vi "Tree.vi"() -> ()   [LabVIEW 2013]
panel:
  in  "全收回":bool
  in  "全展开":bool
  in  "新建项目":bool
  out "当前油动机":string
  out "当前项目":string
  in  "新建油动机":bool
  in  "刷新":bool
  in  "stop":bool
  in  "Path":path
  in  "Tree":string(tree)
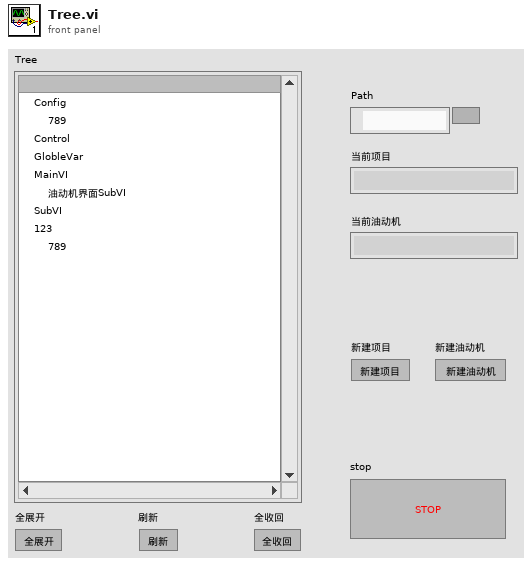
[diagram p1: front panel]
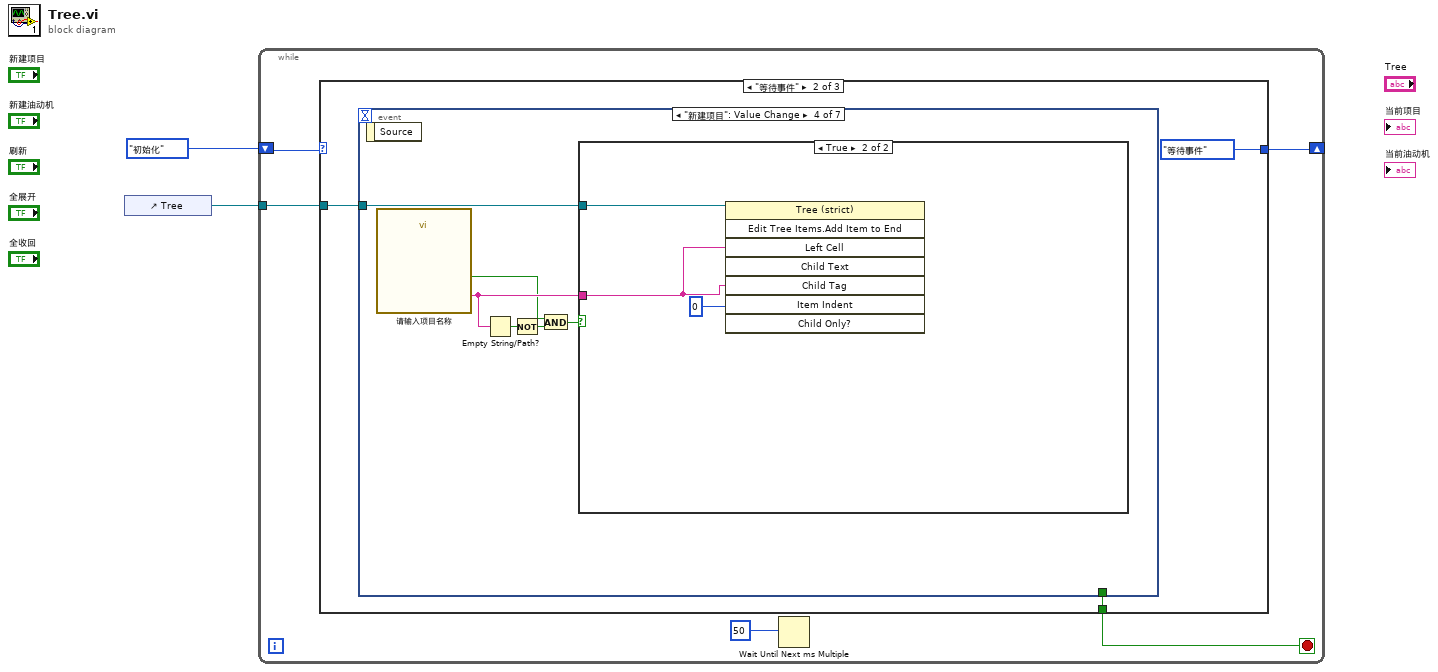
[diagram p0: block diagram]
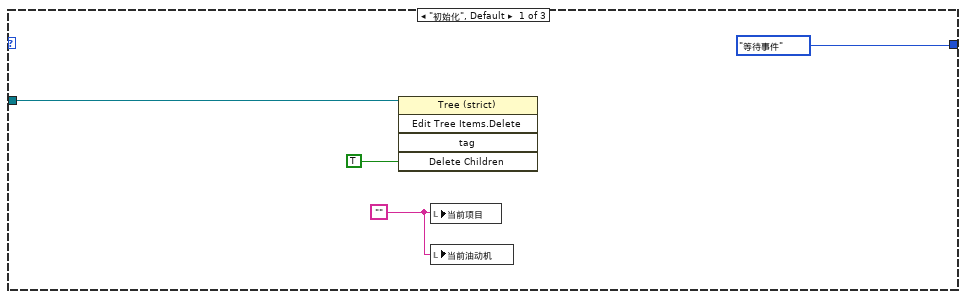
[diagram p2: hidden frame]
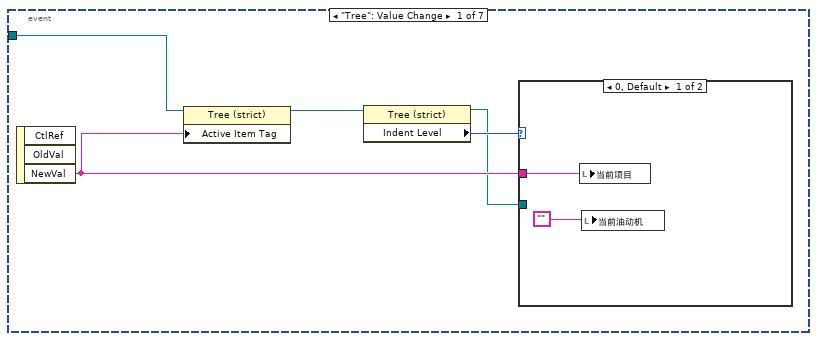
[diagram p3: hidden frame]
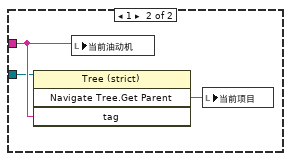
[diagram p4: hidden frame]
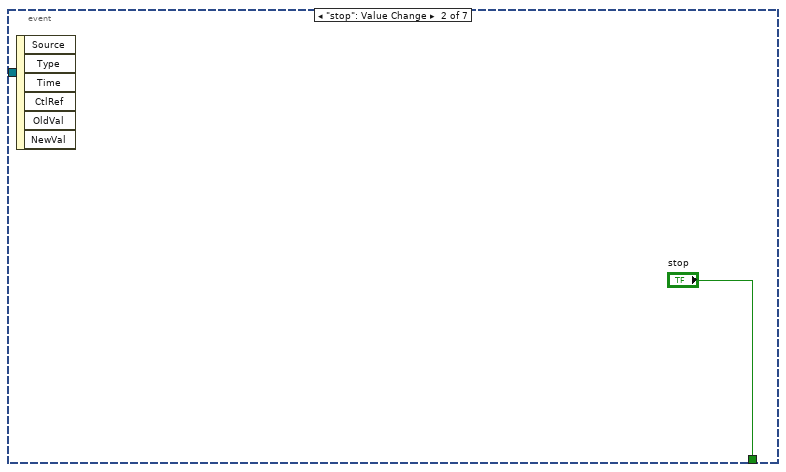
[diagram p5: hidden frame]
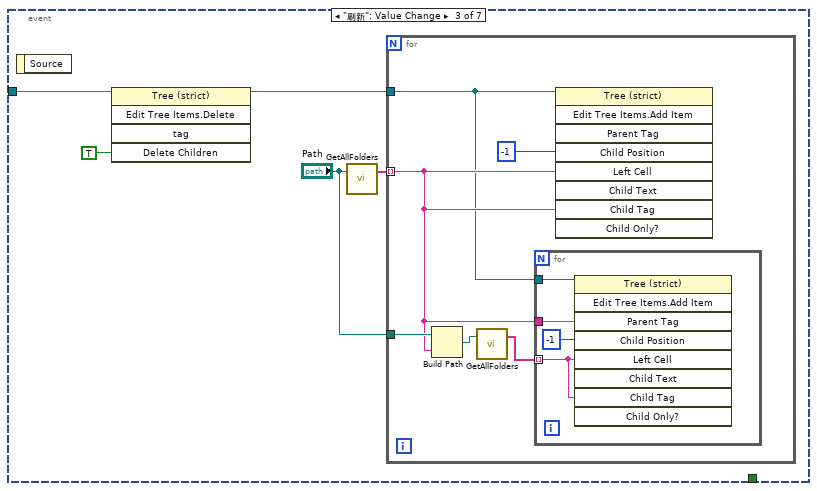
[diagram p6: hidden frame]
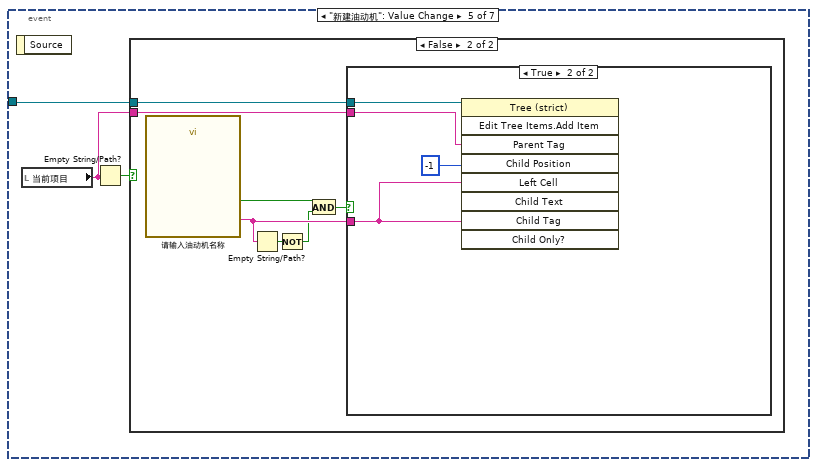
[diagram p8: hidden frame]
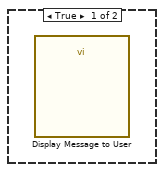
[diagram p9: hidden frame]
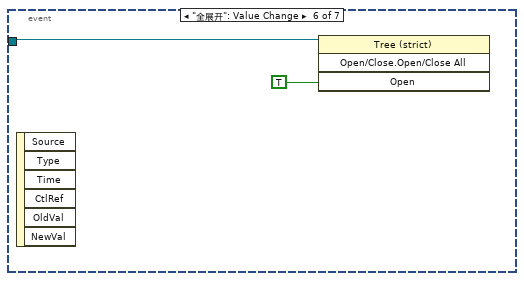
[diagram p11: hidden frame]
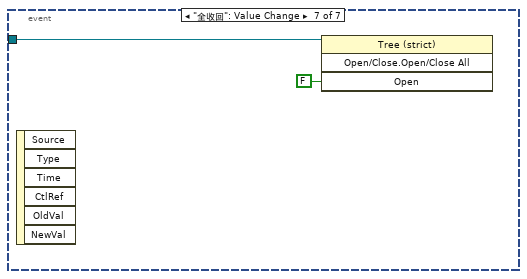
[diagram p12: hidden frame]
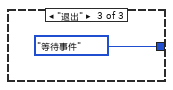
[diagram p13: hidden frame]
diagram:
  n1 = control-ref of="Tree"() -> (w2:refnum<vi>)
  n2 = while {
    tunnel: w2 -> [w6]
    shift-right: [w4] -> _
    shift-left: enum16{"初始化", "等待事件", "退出"}."初始化" -> [w5]
    stop <- w3 stop-if-true
    n3 = case shown="\"等待事件\"" w5 {
      tunnel: [enum16{"初始化", "等待事件", "退出"}."等待事件" enum16{"初始化", "等待事件", "退出"}."等待事件" enum16{"初始化", "等待事件", "退出"}."等待事件"] -> w4
      tunnel: w6 -> [w10 w14 _]
      tunnel: [_ w12 _] -> w3
      frame "初始化", Default {
        w8 = ""
        n4 = invoke class="Tree (strict)" method="Edit Tree Items.Delete"(reference=w10, "Delete Children"=TRUE) -> ()  [unwired: 3 in, 5 out]
        n5 = local write "当前项目"(w8) -> ()
        n6 = local write "当前油动机"(w8) -> ()
      }
      frame "等待事件" {
        n7 = event shown="[3] \"新建项目\": Value Change" {
          selector: _ -> [_ _ _ _ _ _ _]
          dyn-events: _ -> [_ _ _ _ _ _ _]
          timeout: _ -> [_ _ _ _ _ _ _]
          tunnel: w14 -> [w19 _ w27 w46 w52 w65 w67]
          tunnel: [_ "stop" _ _ _ _ _] -> w12
          event "Tree": Value Change {
            n8 = event-data() -> ("NewVal"=w16:string)  [unwired: 1 in, 2 out]
            n9 = property class="Tree (strict)"(reference=w19, "Active Item Tag"=w16) -> (reference out=w18:refnum<vi>)  [unwired: 1 in, 1 out]
            n10 = property class="Tree (strict)"(reference=w18) -> (reference out=w15:refnum<vi>, "Indent Level"=w17:i32)  [unwired: 1 in, 1 out]
            n11 = case shown="0, Default" w17 {
              tunnel: w16 -> [w21 w24]
              tunnel: w15 -> [_ w22]
              frame 0, Default {
                n12 = local write "当前项目"(w21) -> ()
                n13 = local write "当前油动机"("") -> ()
              }
              frame 1 {
                n14 = invoke class="Tree (strict)" method="Navigate Tree.Get Parent"(reference=w22, "tag"=w24) -> ("Navigate Tree:Get Parent"=w23:string)  [unwired: 2 in, 3 out]
                n15 = local write "当前油动机"(w24) -> ()
                n16 = local write "当前项目"(w23) -> ()
              }
            }
          }
          event "stop": Value Change {
            n17 = event-data() -> ()  [unwired: 1 in, 6 out]
          }
          event "刷新": Value Change {
            n18 = event-data() -> ()  [unwired: 1 in, 1 out]
            n19 = invoke class="Tree (strict)" method="Edit Tree Items.Delete"(reference=w27, "Delete Children"=TRUE) -> (reference out=w29:refnum<vi>)  [unwired: 3 in, 4 out]
            n20 = call "GetAllFolders.vi"("FolderPath"="Path") -> ("Folders"=w30:string[])  [unwired: 1 in, 1 out]
            n21 = for {
              tunnel: w30 -> [w32] mode=indexing
              tunnel: w29 -> [w31]
              tunnel: "Path" -> [w35]
              n22 = Build Path(base path=w35, name or relative path=w32) -> (appended path=w34:path)
              n23 = call "GetAllFolders.vi"("FolderPath"=w34) -> ("Folders"=w33:string[])  [unwired: 1 in, 1 out]
              n24 = for {
                tunnel: w33 -> [w40] mode=indexing
                tunnel: w32 -> [w39]
                tunnel: w31 -> [w37]
                n25 = invoke class="Tree (strict)" method="Edit Tree Items.Add Item"(reference=w37, "Parent Tag"=w39, "Child Position"=-1, "Left Cell"=w40, "Child Tag"=w40) -> ()  [unwired: 4 in, 9 out]
              }
              n26 = invoke class="Tree (strict)" method="Edit Tree Items.Add Item"(reference=w31, "Child Position"=-1, "Left Cell"=w32, "Child Tag"=w32) -> ()  [unwired: 5 in, 9 out]
            }
          }
          event "新建项目": Value Change {
            n27 = event-data() -> ()  [unwired: 1 in, 1 out]
            n28 = call "请输入项目名称"() -> ("项目名称"=w45:string, "确认"=w43:bool)  [unwired: 17 in, 1 out]
            n29 = Empty String/Path?(string/path=w45) -> (empty?=w42:bool)
            n30 = Not(x=w42) -> (.not. x?=w41:bool)
            n31 = And(x=w43, y=w41) -> (x .and. y?=w44:bool)
            n32 = case shown="True" w44 {
              tunnel: w46 -> [_ w49]
              tunnel: w45 -> [_ w48]
              frame False {
              }
              frame True {
                n33 = invoke class="Tree (strict)" method="Edit Tree Items.Add Item to End"(reference=w49, "Left Cell"=w48, "Child Tag"=w48, "Item Indent"=0) -> ()  [unwired: 4 in, 8 out]
              }
            }
          }
          event "新建油动机": Value Change {
            n34 = event-data() -> ()  [unwired: 1 in, 1 out]
            n35 = local read "当前项目"() -> (w50:string)
            n36 = Empty String/Path?(string/path=w50) -> (empty?=w51:bool)
            n37 = case shown="False" w51 {
              tunnel: w52 -> [_ w59]
              tunnel: w50 -> [_ w58]
              frame True {
                n38 = call "Display Message to User"() -> ()  [unwired: 10 in, 2 out]
              }
              frame False {
                n39 = call "请输入油动机名称"() -> ("油动机名称"=w57:string, "确认"=w53:bool)  [unwired: 17 in, 1 out]
                n40 = Empty String/Path?(string/path=w57) -> (empty?=w55:bool)
                n41 = Not(x=w55) -> (.not. x?=w54:bool)
                n42 = And(x=w53, y=w54) -> (x .and. y?=w56:bool)
                n43 = case shown="True" w56 {
                  tunnel: w59 -> [_ w62]
                  tunnel: w57 -> [_ w61]
                  tunnel: w58 -> [_ w60]
                  frame False {
                  }
                  frame True {
                    n44 = invoke class="Tree (strict)" method="Edit Tree Items.Add Item"(reference=w62, "Parent Tag"=w60, "Child Position"=-1, "Left Cell"=w61, "Child Tag"=w61) -> ()  [unwired: 4 in, 9 out]
                  }
                }
              }
            }
          }
          event "全展开": Value Change {
            n45 = event-data() -> ()  [unwired: 1 in, 6 out]
            n46 = invoke class="Tree (strict)" method="Open/Close.Open/Close All"(reference=w65, "Open"=TRUE) -> ()  [unwired: 2 in, 4 out]
          }
          event "全收回": Value Change {
            n47 = event-data() -> ()  [unwired: 1 in, 6 out]
            n48 = invoke class="Tree (strict)" method="Open/Close.Open/Close All"(reference=w67, "Open"=FALSE) -> ()  [unwired: 2 in, 4 out]
          }
        }
      }
      frame "退出" {
      }
    }
    n49 = Wait Until Next ms Multiple(millisecond multiple=50) -> ()  [unwired: 1 out]
  }
